vi "Error Log(by Ref) Example.vi"() -> ()   [LabVIEW 2017]
doc: "Demonstrates how to use the Error Log API (by Reference)."
uses:
  <vilib>/BenjaminR/Error Log/Serializer/Type Defs/Display Format.ctl
  <vilib>/BenjaminR/Error Log/Handler.UserEvent.Console/Handler.UserEvent.Console.lvclass
  C:/Program Files (x86)/National Instruments/LabVIEW 2017/vi.lib/BenjaminR/Error Log/Handler/Handler.lvclass
  <vilib>/BenjaminR/Error Log/Handler.File.Text/Handler.File.Text.lvclass
  <vilib>/BenjaminR/Error Log/Logger/Logger.lvclass
  <vilib>/BenjaminR/Error Log/Serializer/Serializer.lvlib
panel:
  in  "Name":string(combo)
  in  "Logger Display Format":T1=enum."PlainText.INI"
  in  "Logger Name":string="Logger Example"
  in  "Erase":bool
  in  "Show Console":bool
  in  "Error Level":T2(ring)
  in  "Error Message":string="Error log message."
  in  "Error":errorcluster={"status"=TRUE, "code"=5000, "source"="My Error Code"}
  in  "Send Error":bool
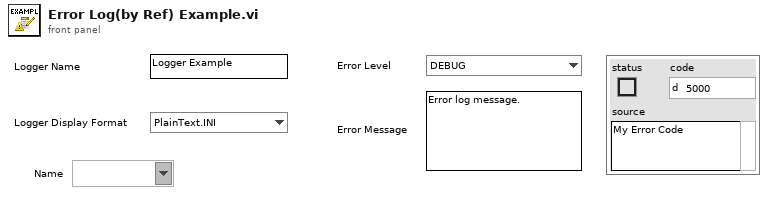
[diagram p1: front panel]
types:
  T1 = typedef "Serializer.lvlib/Display Format.ctl" = enum16{"PlainText", "PlainText.INI", "XML", "JSON"}
  T2 = enum16{"DEBUG", "INFO", "WARNING", "ERROR", "CRITICAL"}
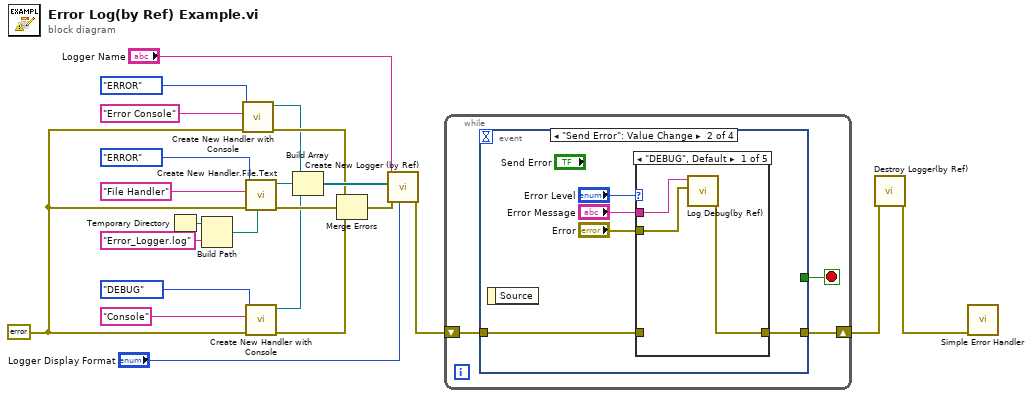
[diagram p0: block diagram]
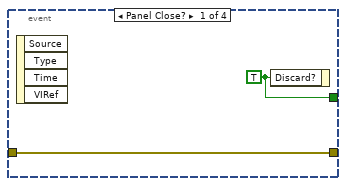
[diagram p2: hidden frame]
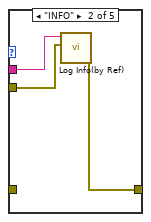
[diagram p3: hidden frame]
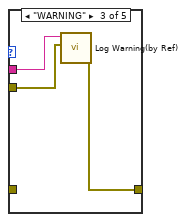
[diagram p4: hidden frame]
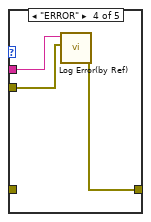
[diagram p5: hidden frame]
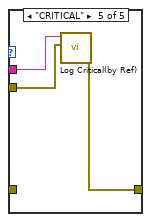
[diagram p6: hidden frame]
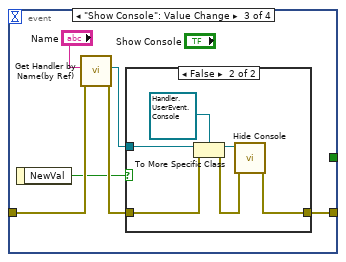
[diagram p7: hidden frame]
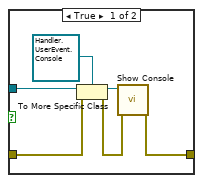
[diagram p8: hidden frame]
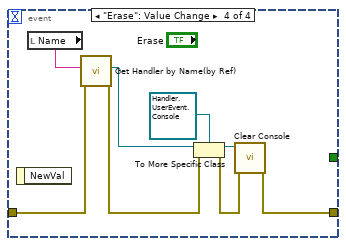
[diagram p9: hidden frame]
diagram:
  w5 = errorcluster {"status"=FALSE, "code"=0, "source"=""} ("error in (no error)")
  n1 = Temporary Directory() -> (w14:path)
  n2 = Build Path(base path=w14, name or relative path="Error_Logger.log") -> (appended path=w12:path)
  n3 = call <vilib>:"Create New Handler with Console.vi"("error in (no error)"=w5, "Name"="Error Console", "Level"=T2."ERROR") -> ("error out"=w4:errorcluster, "Handler.UserEvent.Console out"=w1:refnum<class "Handler.UserEvent.Console.lvclass">)  [unwired: 7 in]
  n4 = call <vilib>:"Create New Handler.File.Text.vi"("File Path"=w12, "error in (no error)"=w5, "Name"="File Handler", "Level"=T2."ERROR") -> ("error out"=w23:errorcluster, "Handler.File.Text out"=w22:refnum<class "Handler.File.Text.lvclass">)  [unwired: 6 in]
  n5 = call <vilib>:"Create New Handler with Console.vi"("error in (no error)"=w5, "Name"="Console", "Level"=T2."DEBUG") -> ("error out"=w11:errorcluster, "Handler.UserEvent.Console out"=w21:refnum<class "Handler.UserEvent.Console.lvclass">)  [unwired: 7 in]
  n6 = Build Array(w1, w22, w21) -> (w20:refnum<class "Handler.lvclass">[])
  n7 = Merge Errors(w4, w23, w11) -> (w19:errorcluster)
  n8 = call <vilib>:"Create New Logger (by Ref).vi"("Display Format"="Logger Display Format", "error in (no error)"=w19, "Handlers"=w20, "Name"="Logger Name") -> ("error out"=w10:errorcluster)  [unwired: 7 in]
  n9 = while {
    shift-right: [w24] -> w9
    shift-left: w10 -> [w25]
    stop <- w26 stop-if-true
    n10 = event shown="[1] \"Send Error\": Value Change" {
      selector: _ -> [_ _ _ _]
      dyn-events: _ -> [_ _ _ _]
      timeout: _ -> [_ _ _ _]
      tunnel: [w28 _ _ _] -> w26
      tunnel: w25 -> [w27 w32 w54 w74]
      tunnel: [w27 w29 w51 w71] -> w24
      event Panel Close? {
        w28 = TRUE ("Discard?")
        n11 = event-data() -> ()  [unwired: 1 in, 4 out]
        n12 = event-data("Discard?"=w28) -> ()  [unwired: 1 in, 1 out]
      }
      event "Send Error": Value Change {
        n13 = event-data() -> ()  [unwired: 1 in, 1 out]
        n14 = case shown="\"DEBUG\", Default" "Error Level" {
          tunnel: w32 -> [_ _ _ _ _]
          tunnel: "Error Message" -> [w34 w39 w41 w44 w47]
          tunnel: "Error" -> [w35 w38 w42 w45 w48]
          tunnel: [w36 w37 w40 w43 w46] -> w29
          frame "DEBUG", Default {
            n15 = call <vilib>:"Log Debug(by Ref).vi"("error in (no error)"=w35, "Message"=w34) -> ("error out"=w36:errorcluster)  [unwired: 9 in]
          }
          frame "INFO" {
            n16 = call <vilib>:"Log Info(by Ref).vi"("error in (no error)"=w38, "Message"=w39) -> ("error out"=w37:errorcluster)  [unwired: 9 in]
          }
          frame "WARNING" {
            n17 = call <vilib>:"Log Warning(by Ref).vi"("error in (no error)"=w42, "Message"=w41) -> ("error out"=w40:errorcluster)  [unwired: 9 in]
          }
          frame "ERROR" {
            n18 = call <vilib>:"Log Error(by Ref).vi"("error in (no error)"=w45, "Message"=w44) -> ("error out"=w43:errorcluster)  [unwired: 9 in]
          }
          frame "CRITICAL" {
            n19 = call <vilib>:"Log Critical(by Ref).vi"("error in (no error)"=w48, "Message"=w47) -> ("error out"=w46:errorcluster)  [unwired: 9 in]
          }
        }
      }
      event "Show Console": Value Change {
        n20 = event-data() -> ("NewVal"=w50:bool)  [unwired: 1 in]
        n21 = call <vilib>:"Get Handler by Name(by Ref).vi"("error in (no error)"=w54, "Handler Name"="Name") -> ("error out"=w52:errorcluster, "Handler"=w53:refnum<class "Handler.lvclass">)  [unwired: 8 in]
        n22 = case shown="False" w50 {
          tunnel: w53 -> [w60 w66]
          tunnel: w52 -> [w57 w63]
          tunnel: [w55 w61] -> w51
          frame True {
            n23 = To More Specific Class(target class=refnum<class "Handler.UserEvent.Console.lvclass"> refnum ("Error Log.lvlib:Handler.UserEvent.Console.lvclass"), reference=w60, error in=w57) -> (specific class reference=w59:refnum<class "Handler.UserEvent.Console.lvclass">, error out=w56:errorcluster)
            n24 = call <vilib>:"Show Console.vi"("error in (no error)"=w56, "Handler.UserEvent.Console in"=w59) -> ("error out"=w55:errorcluster)  [unwired: 8 in, 1 out]
          }
          frame False {
            n25 = To More Specific Class(target class=refnum<class "Handler.UserEvent.Console.lvclass"> refnum ("Error Log.lvlib:Handler.UserEvent.Console.lvclass"), reference=w66, error in=w63) -> (specific class reference=w65:refnum<class "Handler.UserEvent.Console.lvclass">, error out=w62:errorcluster)
            n26 = call <vilib>:"Hide Console.vi"("error in (no error)"=w62, "Handler.UserEvent.Console in"=w65) -> ("error out"=w61:errorcluster)  [unwired: 8 in, 1 out]
          }
        }
      }
      event "Erase": Value Change {
        n27 = event-data() -> ()  [unwired: 1 in, 1 out]
        n28 = local read "Name"() -> (w67:string)
        n29 = call <vilib>:"Get Handler by Name(by Ref).vi"("error in (no error)"=w74, "Handler Name"=w67) -> ("error out"=w72:errorcluster, "Handler"=w73:refnum<class "Handler.lvclass">)  [unwired: 8 in]
        n30 = To More Specific Class(target class=refnum<class "Handler.UserEvent.Console.lvclass"> refnum ("Error Log.lvlib:Handler.UserEvent.Console.lvclass"), reference=w73, error in=w72) -> (specific class reference=w70:refnum<class "Handler.UserEvent.Console.lvclass">, error out=w68:errorcluster)
        n31 = call <vilib>:"Clear Console.vi"("error in (no error)"=w68, "Handler.UserEvent.Console in"=w70) -> ("error out"=w71:errorcluster)  [unwired: 8 in, 1 out]
      }
    }
  }
  n32 = call <vilib>:"Destroy Logger(by Ref).vi"("error in (no error)"=w9) -> ("error out"=w8:errorcluster)  [unwired: 10 in]
  n33 = call <vilib>:"Simple Error Handler.vi"("error in (no error)"=w8) -> ()  [unwired: 4 in, 5 out]
